vi "LINX TCP Benchmark.vi"() -> ()   [LabVIEW 2013]
uses:
  <vilib>/ptbypt/NI_PtbyPt.lvlib
panel:
  out "Loop Time vs Packet Size - WIFI":dbl(graph)
  out "Failed Packets":i32
  out "Iteration":i32
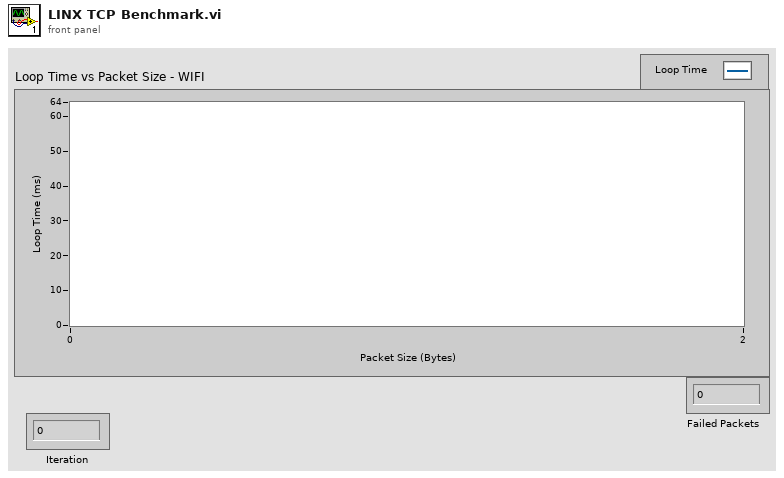
[diagram p1: front panel]
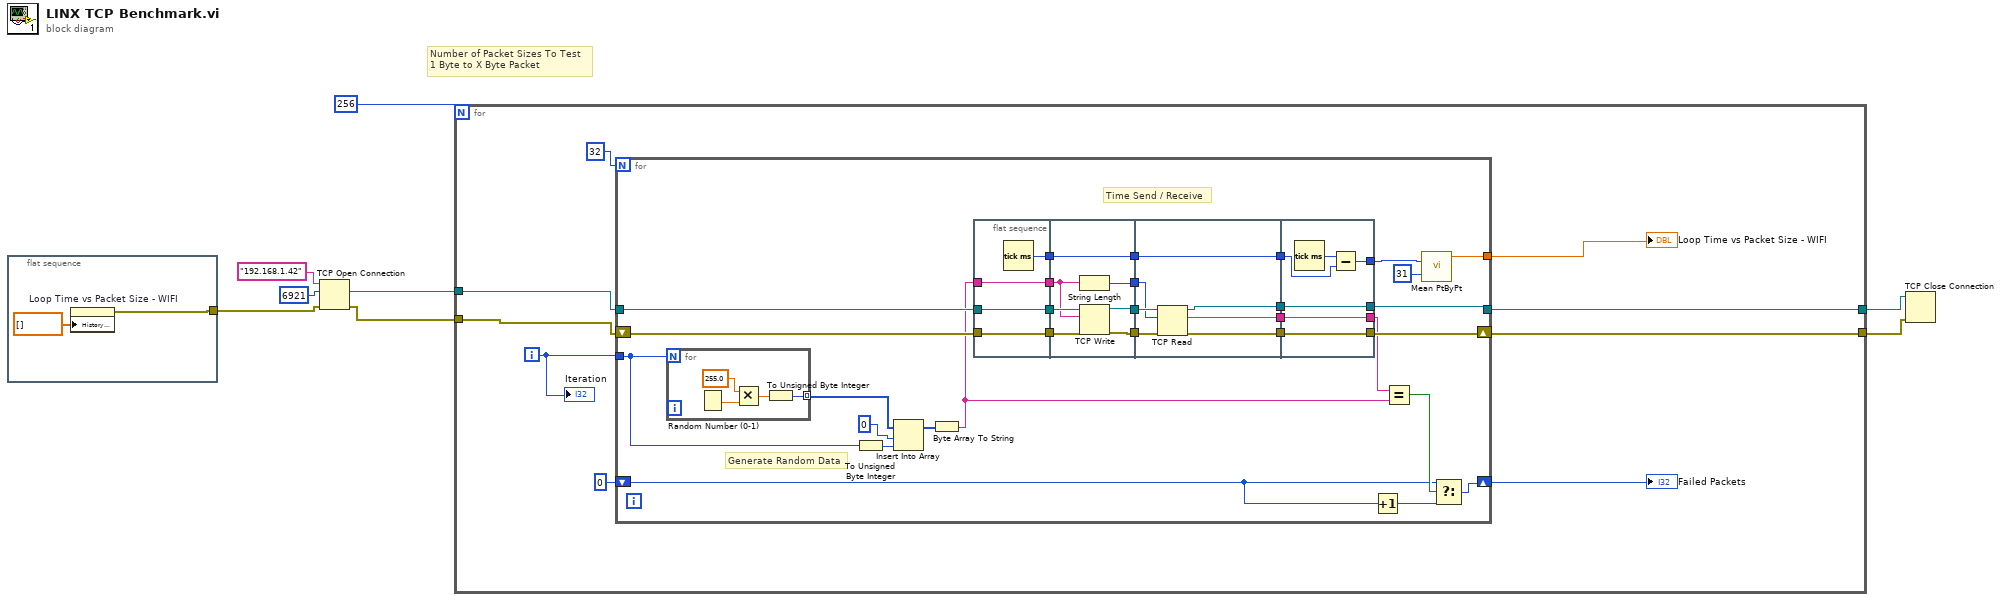
[diagram p0: block diagram]
diagram:
  # "Number of Packet Sizes To Test\n1 Byte to X Byte Packet"
  n1 = flat-sequence {
    tunnel: [w9] -> w5
    frame #0 {
      n2 = property on="Loop Time vs Packet Size - WIFI" class="WFChart (strict)"("History Data"=dbl[] []) -> (error out=w9:errorcluster)  [unwired: 2 in, 1 out]
    }
  }
  n3 = TCP Open Connection(address="192.168.1.42", remote port or service name=u16 6921, error in (no error)=w5) -> (connection ID=w1:refnum<k5>, error out=w4:errorcluster)  [unwired: 2 in]
  n4 = for {
    N: 256 -> [_]
    tunnel: w4 -> [w14]
    tunnel: [w13] -> w3
    tunnel: [w12] -> w2
    tunnel: w1 -> [w11]
    i -> [w15]
    n5 = for {
      N: 32 -> [_]
      tunnel: w11 -> [w48]
      shift-right: [w41] -> w12
      shift-left: w14 -> [w49]
      tunnel: [w36] -> w13
      shift-right: [w27] -> w18
      shift-left: 0 -> [w28]
      tunnel: [w26] -> w17
      tunnel: w15 -> [w22]
      # "Time Send / Receive"
      # "Generate Random Data"
      n6 = for {
        N: w22 -> [_]
        tunnel: [w50] -> w24 mode=indexing
        n7 = Random Number (0-1)() -> (number: 0 to 1=w53:dbl)
        n8 = Multiply(x=255.0, y=w53) -> (x*y=w51:dbl)
        n9 = To Unsigned Byte Integer(number=w51) -> (unsigned 8bit integer=w50:u8)
      }
      n10 = To Unsigned Byte Integer(number=w22) -> (unsigned 8bit integer=w21:u8)
      n11 = Insert Into Array(array=w24, index=0, new element=w21) -> (w23:u8[])
      n12 = Byte Array To String(unsigned byte array=w23) -> (string=w25:string)
      n13 = flat-sequence {
        tunnel: w48 -> [w56]
        tunnel: w49 -> [w57]
        tunnel: [w57] -> w44
        tunnel: [w56] -> w43
        tunnel: [w55] -> w40
        tunnel: [w54] -> w33
        tunnel: w25 -> [w54]
        tunnel: [w64] -> w47
        tunnel: [w63] -> w46
        tunnel: [w62] -> w45
        tunnel: w44 -> [w61]
        tunnel: w43 -> [w60]
        tunnel: w40 -> [w59]
        tunnel: [w59] -> w39
        tunnel: w33 -> [w58]
        tunnel: w47 -> [w71]
        tunnel: w46 -> [w69]
        tunnel: w45 -> [w70]
        tunnel: [w68] -> w42
        tunnel: w39 -> [w67]
        tunnel: [w67] -> w38
        tunnel: [w66] -> w37
        tunnel: [w65] -> w31
        tunnel: [w77] -> w41
        tunnel: w42 -> [w77]
        tunnel: w38 -> [w75]
        tunnel: w37 -> [w74]
        tunnel: [w74] -> w36
        tunnel: [w73] -> w35
        tunnel: [w72] -> w32
        tunnel: w31 -> [w72]
        frame #0 {
          n14 = Tick Count (ms)() -> (millisecond timer value=w55:u32)
        }
        frame #1 {
          n15 = String Length(string=w58) -> (length=w62:i32)
          n16 = TCP Write(connection ID=w60, data in=w58, error in (no error)=w61) -> (connection ID out=w64:refnum<k5>, error out=w63:errorcluster)  [unwired: 1 in, 1 out]
        }
        frame #2 {
          n17 = TCP Read(connection ID=w71, bytes to read=w70, error in (no error)=w69) -> (connection ID out=w66:refnum<k5>, data out=w65:string, error out=w68:errorcluster)  [unwired: 2 in]
        }
        frame #3 {
          n18 = Tick Count (ms)() -> (millisecond timer value=w76:u32)
          n19 = Subtract(x=w76, y=w75) -> (x-y=w73:u32)
        }
      }
      n20 = Increment(x=w28) -> (x+1=w29:i32)
      n21 = Equal?(x=w32, y=w25) -> (x = y?=w30:bool)
      n22 = call <vilib>:"Mean PtByPt.vi"("x"=w35, "sample length"=31) -> ("mean"=w26:dbl)  [unwired: 2 in, 1 out]
      n23 = Select(t=w28, s=w30, f=w29) -> (s? t:f=w27:i32)
    }
    "Failed Packets" <- w18
    "Loop Time vs Packet Size - WIFI" <- w17
    "Iteration" <- w15
  }
  n24 = TCP Close Connection(connection ID=w3, error in (no error)=w2) -> ()  [unwired: 1 in, 2 out]
